vi "UpdateDataDisPanel.vi"(0 "Input String":string, 1 "send/read":bool=TRUE, 2 "Display Style":u32, 3 "error in":errorcluster, 4 "Clear Screen":bool) -> (6 "Output String":string, 7 "error out":errorcluster)   [LabVIEW 2023]
panel:
  out "Data Stream":string
  out "time string":string
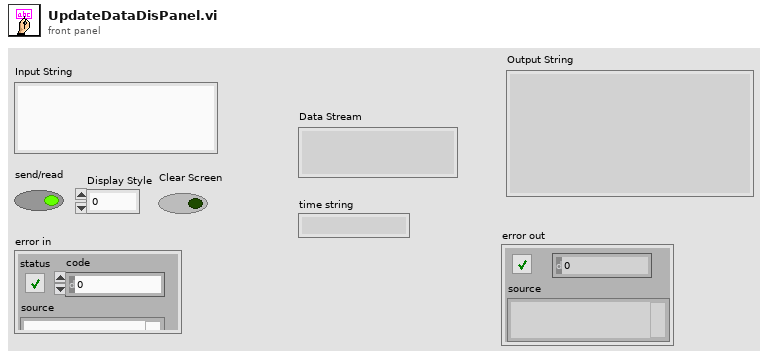
[diagram p1: front panel]
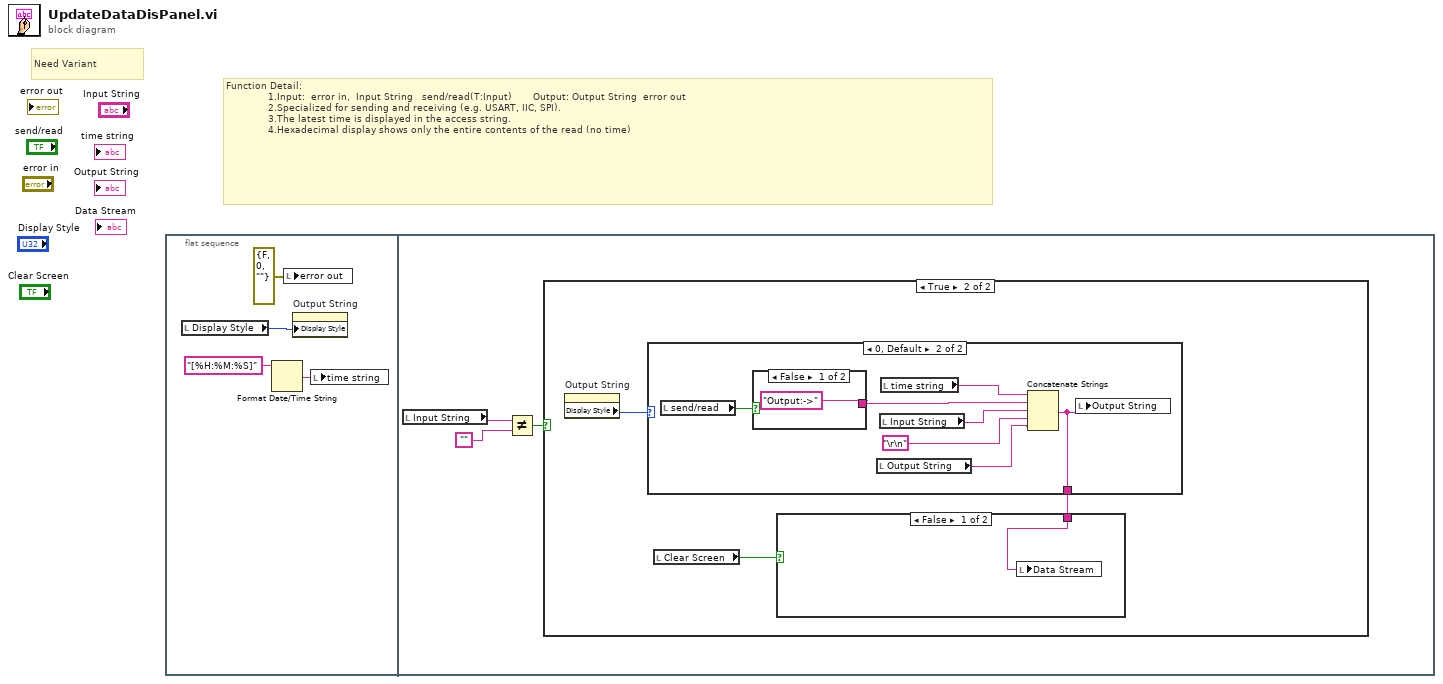
[diagram p0: block diagram]
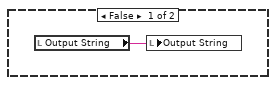
[diagram p2: hidden frame]
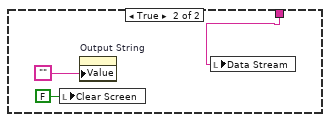
[diagram p3: hidden frame]
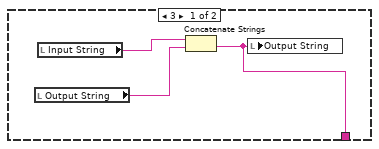
[diagram p4: hidden frame]
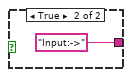
[diagram p5: hidden frame]
diagram:
  # "Function Detail:\n              1.Input:  error in,  Input String   send/read(T:Input)       Output: Output String  error out\n              2.Specialized for sending and receiving (e.g. USART, IIC, SPI).\n              3.The latest time is displayed in the access string.\n              4.Hexadecimal display shows only the entire contents of the read (no time)"
  # "Need Variant"
  n1 = flat-sequence {
    frame #0 {
      n2 = local read "Display Style"() -> (w2:u32)
      n3 = Format Date/Time String(time format string (%c)="[%H:%M:%S]") -> (date/time string=w4:string)  [unwired: 2 in]
      n4 = local write "error out"(errorcluster {"status"=FALSE, "code"=0, "source"=""} ("error out")) -> ()
      n5 = property on="Output String" class="Str"("Display Style"=w2) -> ()  [unwired: 2 in, 2 out]
      n6 = local write "time string"(w4) -> ()
    }
    frame #1 {
      n7 = local read "Input String"() -> (w7:string)
      n8 = Not Equal?(x=w7, y="") -> (x != y?=w5:bool)
      n9 = case shown="True" w5 {
        frame False {
          n10 = local read "Output String"() -> (w8:string)
          n11 = local write "Output String"(w8) -> ()
        }
        frame True {
          n12 = property on="Output String" class="Str"() -> ("Display Style"=w11:u32)  [unwired: 2 in, 2 out]
          n13 = case shown="0, Default" w11 {
            tunnel: [w16 w19] -> w9
            frame 3 {
              n14 = local read "Output String"() -> (w17:string)
              n15 = local read "Input String"() -> (w18:string)
              n16 = Concatenate Strings(w18, w17) -> (w16:string)
              n17 = local write "Output String"(w16) -> ()
            }
            frame 0, Default {
              n18 = local read "send/read"() -> (w21:bool)
              n19 = case shown="False" w21 {
                tunnel: ["Output:->" ("string") "Input:->" ("string")] -> w20
                frame False {
                }
                frame True {
                }
              }
              n20 = local read "Output String"() -> (w22:string)
              n21 = local read "Input String"() -> (w25:string)
              n22 = local read "time string"() -> (w23:string)
              n23 = Concatenate Strings(w23, w20, w25, "\r\n", w22) -> (w19:string)
              n24 = local write "Output String"(w19) -> ()
            }
          }
          n25 = local read "Clear Screen"() -> (w10:bool)
          n26 = case shown="False" w10 {
            tunnel: w9 -> [w12 w13]
            frame False {
              n27 = local write "Data Stream"(w12) -> ()
            }
            frame True {
              n28 = local write "Clear Screen"(FALSE ("Clear Screen")) -> ()
              n29 = property on="Output String" class="Str"("Value"="") -> ()  [unwired: 2 in, 2 out]
              n30 = local write "Data Stream"(w13) -> ()
            }
          }
        }
      }
    }
  }
